vi "Find Image refnum.vi"(0 "Image to Add refnum [ ]":T3, 5 "Type and run direction":T2=enum."ASCII", 9 "Text cluster":cluster{"Text":string, "Image?":bool}, 11 "error in (no error)":errorcluster) -> (4 "InstanceImage refnum":refnum<k24>, 6 "Find Image?":bool, 8 "Text element type":T1=enum."Not a valid image", 10 "Text Duplicate":string, 15 "error out":errorcluster)   [LabVIEW 2019, in "Exaprom PDF.lvlib"]
doc: "Version 2.0\nDeveloped by Jean-Marc Simard\nCopyright © 2012, Exaprom Inc.\nAll rights reserved.\nLicense: BSD\n\nWith iTextSharp 4.1.6 (http://itextsharp.sourceforge.net)\nunder Mozilla Public License Version 1.1\n(http://www.mozilla.org/MPL/MPL-1.1.html)"
uses:
  Controls/General Controls/Image to Add refnum [ ].ctl
  C:/work/niobrara_lv/labview pdf writer fixing/DLL/itextsharp.dll
  DLL/itextsharp.dll
  Controls/Text Controls/Unicode/Type and run direction.ctl
  Controls/Text Controls/Text element type.ctl
  General/Stop if it True.vi
  Exaprom PDF.lvlib
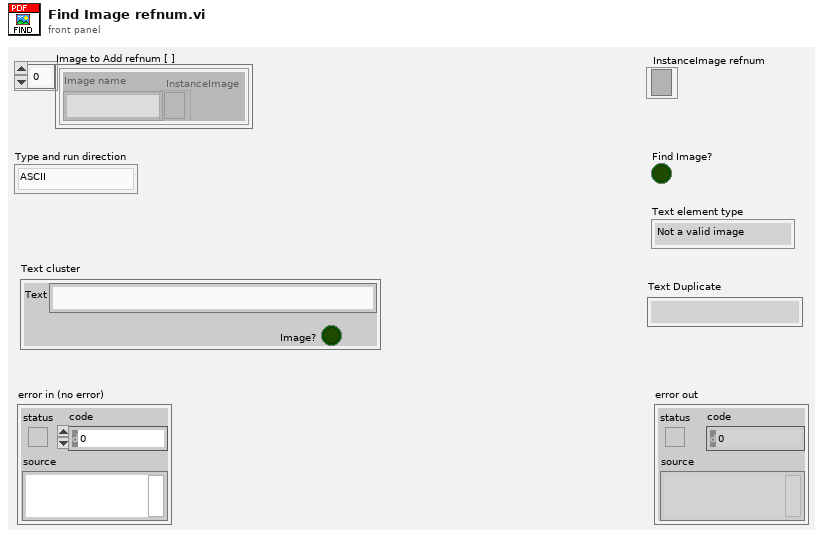
[diagram p1: front panel]
types:
  T1 = typedef "Exaprom PDF.lvlib/Text element type.ctl" = enum16{"Text", "Image", "Not a valid image", "Link"}
  T2 = typedef "Exaprom PDF.lvlib/Type and run direction.ctl" = enum16{"Select", "ASCII", "UTF-16", "UTF-16 (default)", "UTF-16 (LTR)", "UTF-16 (RTL)"}
  T3 = typedef "Exaprom PDF.lvlib/Image to Add refnum [ ].ctl" = cluster{"Image name":string, "InstanceImage":refnum<k24>}[]
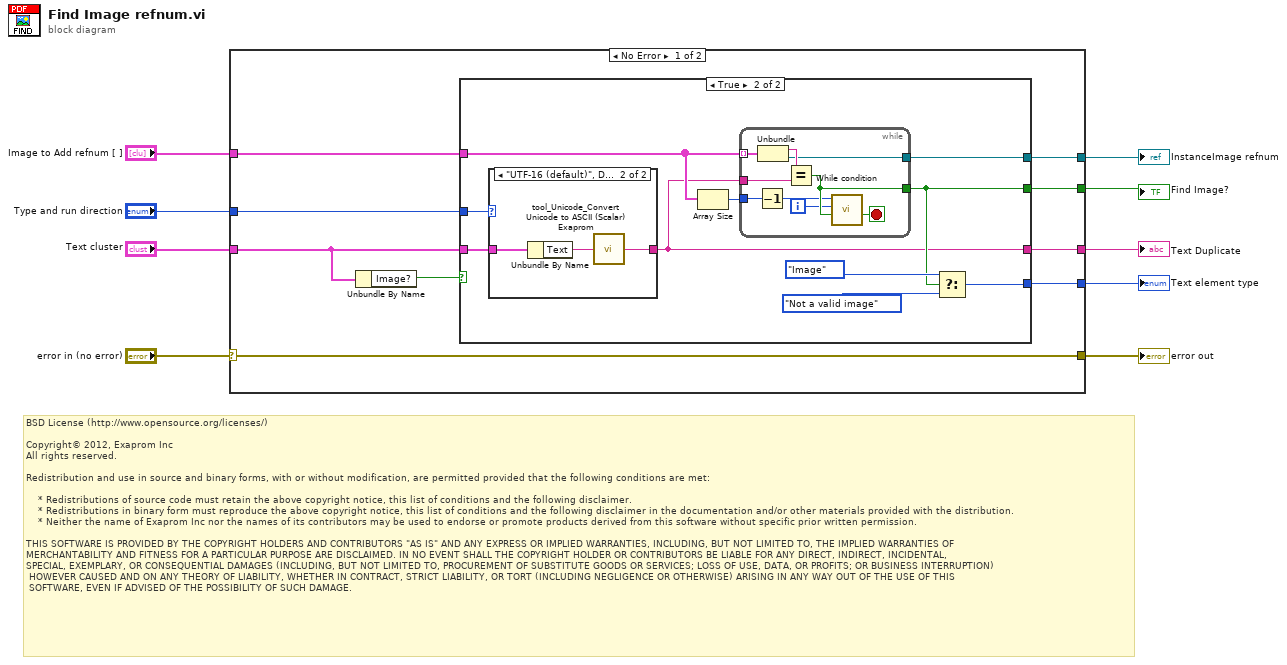
[diagram p0: block diagram]
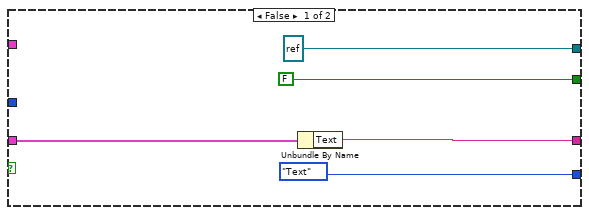
[diagram p2: hidden frame]
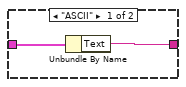
[diagram p3: hidden frame]
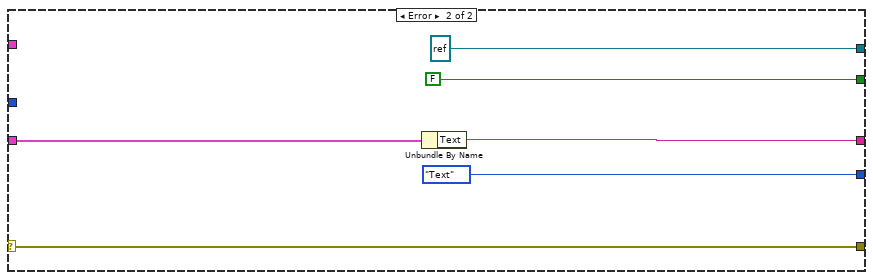
[diagram p4: hidden frame]
diagram:
  # "BSD License (http://www.opensource.org/licenses/)\n\nCopyright© 2012, Exaprom Inc\nAll rights reserved.\n\nRedistribution and use in source and binary forms, with or without modification, are permitted provided that the following conditions are met:\n\n    * Redistributions of source code must retain the above copyright notice, this list of conditions and the following disclaimer.\n    * Redistributions in binary form must reproduce the above copyright notice, this list of conditions and the following disclaimer in the documentation and/or other materials provided with the distribution.\n    * Neither the name of Exaprom Inc nor the names of its contributors may be used to endorse or promote products derived from this software without specific prior written permission.\n\nTHIS SOFTWARE IS PROVIDED BY THE COPYRIGHT HOLDERS AND CONTRIBUTORS \"AS IS\" AND ANY EXPRESS OR IMPLIED WARRANTIES, INCLUDING, BUT NOT LIMITED TO, THE IMPLIED WARRANTIES OF \nMERCHANTABILITY AND FITNESS FOR A PARTICULAR PURPOSE ARE DISCLAIMED. IN NO EVENT SHALL THE COPYRIGHT HOLDER OR CONTRIBUTORS BE LIABLE FOR ANY DIRECT, INDIRECT, INCIDENTAL,\nSPECIAL, EXEMPLARY, OR CONSEQUENTIAL DAMAGES (INCLUDING, BUT NOT LIMITED TO, PROCUREMENT OF SUBSTITUTE GOODS OR SERVICES; LOSS OF USE, DATA, OR PROFITS; OR BUSINESS INTERRUPTION)\n HOWEVER CAUSED AND ON ANY THEORY OF LIABILITY, WHETHER IN CONTRACT, STRICT LIABILITY, OR TORT (INCLUDING NEGLIGENCE OR OTHERWISE) ARISING IN ANY WAY OUT OF THE USE OF THIS\n SOFTWARE, EVEN IF ADVISED OF THE POSSIBILITY OF SUCH DAMAGE."
  n1 = case shown="No Error" "error in (no error)" {
    selector: "error in (no error)" -> [w16 w53]
    tunnel: "Image to Add refnum [ ]" -> [w15 _]
    tunnel: [w17 refnum<k24> refnum ("InstanceImage")] -> w8
    tunnel: [w18 FALSE] -> w7
    tunnel: [w16 w53] -> w5
    tunnel: "Text cluster" -> [w13 w50]
    tunnel: [w12 w48] -> w3
    tunnel: [w11 Text_element_type."Text" ("Text element type")] -> w2
    tunnel: "Type and run direction" -> [w10 _]
    frame No Error {
      n2 = Unbundle By Name(w13) -> ("Image?"=w14:bool)
      n3 = case shown="True" w14 {
        tunnel: [FALSE w26] -> w18
        tunnel: [refnum<k24> refnum ("InstanceImage") w33] -> w17
        tunnel: w15 -> [_ w32]
        tunnel: w13 -> [w23 w29]
        tunnel: [w19 w24] -> w12
        tunnel: [Text_element_type."Text" ("Text element type") w25] -> w11
        tunnel: w10 -> [_ w30]
        frame False {
          n4 = Unbundle By Name(w23) -> ("Text"=w19:string)
        }
        frame True {
          n5 = case shown="\"UTF-16 (default)\", Default" w30 {
            tunnel: w29 -> [w35 w38]
            tunnel: [w34 w36] -> w24
            frame "ASCII" {
              n6 = Unbundle By Name(w35) -> ("Text"=w34:string)
            }
            frame "UTF-16 (default)", Default {
              n7 = Unbundle By Name(w38) -> ("Text"=w37:string)
              n8 = call "tool_Unicode_Convert Unicode to ASCII (Scalar) Exaprom.vi"("Unicode"=w37) -> ("ASCII"=w36:string)  [unwired: 4 in]
            }
          }
          n9 = Array Size(array=w32) -> (size(s)=w31:i32)
          n10 = while {
            tunnel: w32 -> [w47] mode=indexing
            tunnel: w24 -> [w46]
            tunnel: [w44] -> w33
            tunnel: w31 -> [w40]
            tunnel: [w42] -> w26
            i -> [w41]
            stop <- w43 stop-if-true
            n11 = Decrement(x=w40) -> (x-1=w39:i32)
            n12 = Unbundle(w47) -> ("Image name"=w45:string, "InstanceImage"=w44:refnum<k24>)
            n13 = Equal?(x=w45, y=w46) -> (x = y?=w42:bool)
            n14 = call-poly "While condition.vi"("Test"=w42, "i"=w41, "N"=w39) -> ("Action"=w43:bool)  [unwired: 5 out]
          }
          n15 = Select(t=Text_element_type."Image" ("Text element type"), s=w26, f=Text_element_type."Not a valid image" ("Text element type")) -> (s? t:f=w25:T1)
        }
      }
    }
    frame Error {
      n16 = Unbundle By Name(w50) -> ("Text"=w48:string)
    }
  }
  "InstanceImage refnum" <- w8
  "Find Image?" <- w7
  "error out" <- w5
  "Text Duplicate" <- w3
  "Text element type" <- w2
